vi "网分校准.vi"(8 "error in (no error)":errorcluster, 11 "RS in":refnum<class "RS.lvclass">) -> (0 "error out":errorcluster, 3 "RS out":refnum<class "RS.lvclass">)   [LabVIEW 2015, in "RS.lvclass"]
uses:
  RS.lvclass
  network_Global/Global.vi
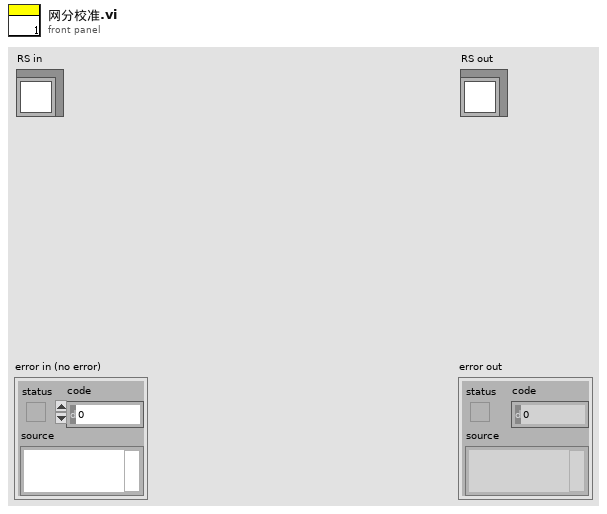
[diagram p1: front panel]
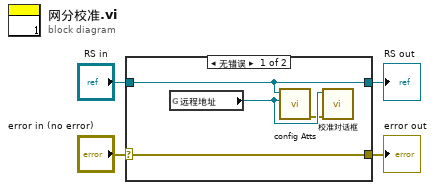
[diagram p0: block diagram]
diagram:
  n1 = case shown="无错误" "error in (no error)" {
    selector: "error in (no error)" -> [w8 w9]
    tunnel: [w8 w9] -> w3
    tunnel: "RS in" -> [w7 w10]
    tunnel: [w7 w10] -> w1
    frame No Error {
      n2 = global read "Global.vi" "远程地址"() -> (w6:refnum<visa-resource-name>)
      n3 = call-dynamic "config Atts.vi"("VISA resource name"=w6, "RS in"=w7) -> ("error out"=w5:errorcluster)  [unwired: 7 in, 2 out]
      n4 = call "校准对话框.vi"("error in"=w5, "RS网分地址"=w6) -> ()  [unwired: 8 in, 2 out]
    }
    frame Error {
    }
  }
  "error out" <- w3
  "RS out" <- w1
